vi "Write Show.vi"(8 "error in (no error)":errorcluster, 10 "Show":bool, 11 "FSM.Annotation in":refnum<class "FSM.Annotation.lvclass">) -> (0 "error out":errorcluster, 3 "FSM.Annotation out":refnum<class "FSM.Annotation.lvclass">)   [LabVIEW 2020, in "FSM.Annotation.lvclass"]
uses:
  FSM.Annotation.lvclass
  FSM.Annotation.lvclass/FSM.Annotation.ctl
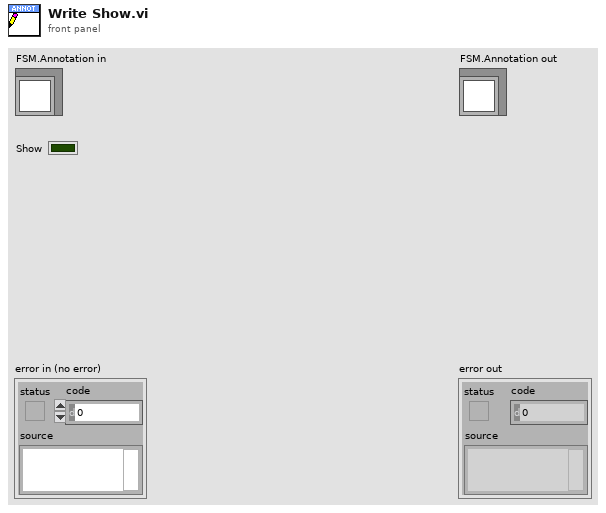
[diagram p1: front panel]
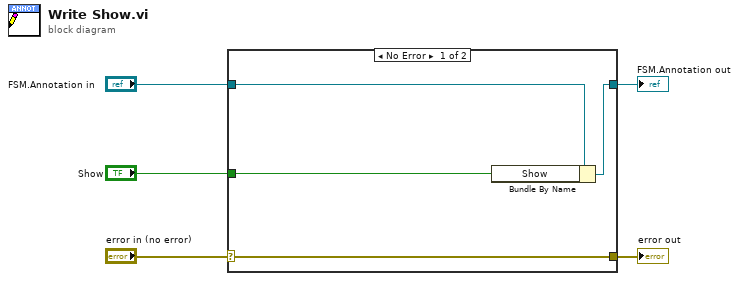
[diagram p0: block diagram]
diagram:
  n1 = case shown="No Error" "error in (no error)" {
    selector: "error in (no error)" -> [w9 w10]
    tunnel: [w9 w10] -> w4
    tunnel: [w7 w11] -> w2
    tunnel: "FSM.Annotation in" -> [w8 w11]
    tunnel: "Show" -> [w6 _]
    frame No Error {
      n2 = Bundle By Name(cluster=w8, "Show"=w6) -> (w7:refnum<class "FSM.Annotation.lvclass">)
    }
    frame Error {
    }
  }
  "error out" <- w4
  "FSM.Annotation out" <- w2
